vi "SCD - Use Global Variables to Compute LCVR Voltages.vi"(2 "error in":errorcluster, 3 "Wavelength (nm)":dbl=557.0 min=0.0 step=0.01 format="%.2f") -> (0 "error out":errorcluster, 1 "Required LCVR Voltages":dbl[](array[numeric])=[1.8374212607235123, 1.6766025168197034, 2.2097290599219055, 2.2205289350684585, 1.959581474179891] format="%.3f")   [LabVIEW 2014]
uses:
  LCVR Voltages Global 2015-Apr-07.vi
panel:
  out "Coefficients":dbl[][](array[numeric])
  out "Final Offsets":dbl[](array[numeric])
  in  "Additional Offsets (nm)":dbl[][](array[numeric])=[[0.0, 0.0, 0.0, 0.0, 0.0, 0.0, 0.0, 0.0, 0.0], [0.0, 0.0, 0.0, 0.0, 0.0, 0.0, 0.0, 0.0, 0.0], [0.0, 0.0, 0.0, 0.0, 0.0, 0.0, 0.0, 0.0, 0.0], [0.0, 0.0, 0.0, 0.0, 0.0, 0.0, 0.0, 0.0, 0.0], [0.0, 0.0, 0.0, 0.0, 0.0, 0.0, 0.0, 0.0, 0.0]] min=-1.0 max=1.0 step=0.005 format="%.4f"
  out "Region Index":i32 caption="min index(es)"
  out "ld (nm)":dbl[](array[numeric])=[782341.3728, 1564132.3776, 3134250.8167000003, 6278016.8802000005, 12632760.0] format="%.5e"
  out "Order":dbl[](array[numeric])=[1404.0, 2808.0, 5627.0, 11271.0, 22680.0]
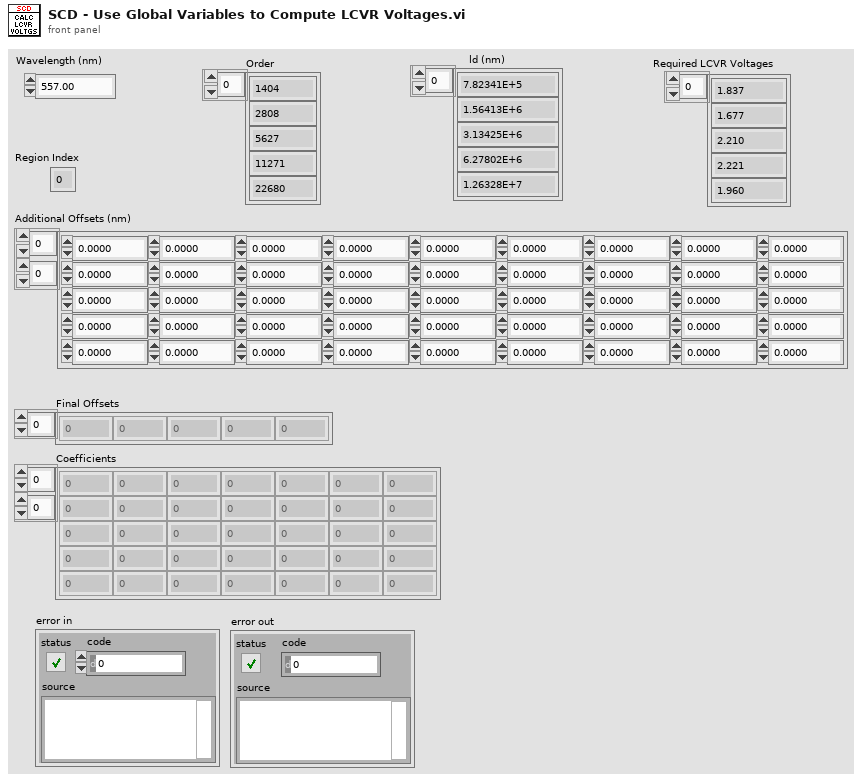
[diagram p1: front panel]
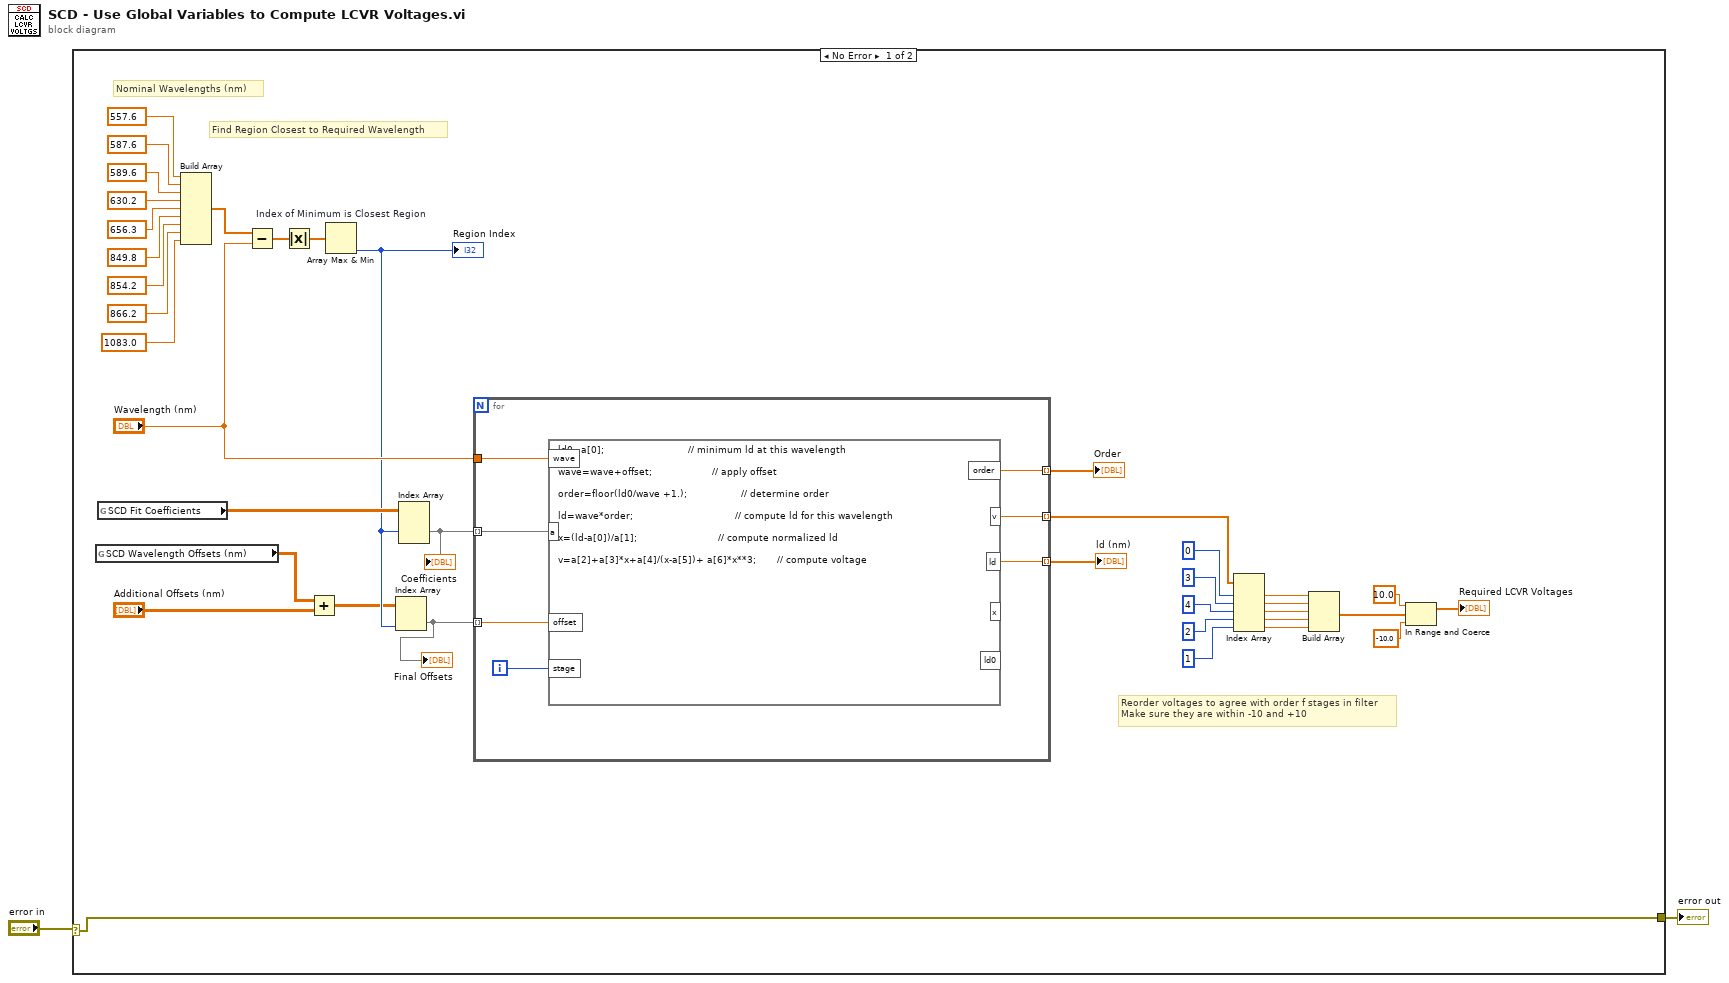
[diagram p0: block diagram]
diagram:
  n1 = case shown="No Error" "error in" {
    selector: "error in" -> [w4 w48]
    tunnel: [w4 w48] -> w1
    frame No Error {
      # "Reorder voltages to agree with order f stages in filter\nMake sure they are within -10 and +10"
      # "Find Region Closest to Required Wavelength"
      # "Nominal Wavelengths (nm)"
      n2 = global read "LCVR Voltages Global 2015-Apr-07.vi" "SCD Wavelength Offsets (nm)"() -> (w26:dbl[][])
      n3 = global read "LCVR Voltages Global 2015-Apr-07.vi" "SCD Fit Coefficients"() -> (w30:dbl[][][])
      n4 = Build Array(557.6 ("element"), 587.6 ("element"), 589.6 ("element"), 630.2 ("element"), 656.3 ("element"), 849.8 ("element"), 854.2 ("element"), 866.2 ("element"), 1083.0 ("element")) -> (w38:dbl[])
      n5 = Subtract(x=w38, y="Wavelength (nm)") -> (x-y=w37:dbl[])
      n6 = Absolute Value(x=w37) -> (abs(x)=w34:dbl[])
      n7 = Add(x=w26, y="Additional Offsets (nm)") -> (x+y=w25:dbl[][])
      n8 = Array Max & Min "Index of Minimum is Closest Region"(array=w34) -> (min index (indices)=w28:i32)  [unwired: 3 out]
      "Region Index" <- w28
      n9 = Index Array(array=w25, index (col)=w28) -> (element=w3:dbl[])  [unwired: 1 in]
      "Final Offsets" <- w3
      n10 = Index Array(array=w30, index (dim 1)=w28) -> (element=w29:dbl[][])  [unwired: 2 in]
      "Coefficients" <- w29
      n11 = for {
        tunnel: [w47] -> w14 mode=indexing
        tunnel: [w46] -> w39 mode=indexing
        tunnel: [w45] -> w40 mode=indexing
        tunnel: "Wavelength (nm)" -> [w43]
        tunnel: w29 -> [w42] mode=indexing
        tunnel: w3 -> [w41] mode=indexing
        i -> [w44]
        n12 = formula code="ld0=a[0];                            // minimum ld at this wavelength\n\nwave=wave+offset;                    // apply offset\n\norder=floor(ld0/wave +1.);                  // determine order\n\nld=wave*order;                                  // compute ld for this wavelength\n\nx=(ld-a[0])/a[1];                           // compute normalized ld\n\nv=a[2]+a[3]*x+a[4]/(x-a[5])+ a[6]*x**3;       // compute voltage"("a"=w42, "wave"=w43, "stage"=w44, "offset"=w41) -> ("order"=w45:dbl, "v"=w47:dbl, "ld"=w46:dbl)  [unwired: 2 out]
      }
      "Order" <- w40
      "ld (nm)" <- w39
      n13 = Index Array(array=w14, index #1=0 ("index"), index #2=3 ("index"), index #3=4 ("index"), index #4=2 ("index"), index #5=1 ("index")) -> (element #1=w13:dbl, element #2=w12:dbl, element #3=w11:dbl, element #4=w10:dbl, element #5=w9:dbl)
      n14 = Build Array(w13, w12, w11, w10, w9) -> (w6:dbl[])
      n15 = In Range and Coerce(upper limit=10.0, x=w6, lower limit=-10.0) -> (coerced(x)=→"Required LCVR Voltages":dbl[])  [unwired: 1 out]
    }
    frame Error {
    }
  }
  "error out" <- w1
